vi "Metric.vi"(5 "Action":enum16{"Init", "Check"}(ring)) -> (2 "Metric?":bool)   [LabVIEW 2011]
uses:
  Globals/SysGlbs.vi
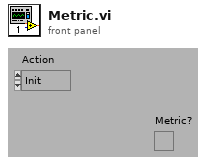
[diagram p1: front panel]
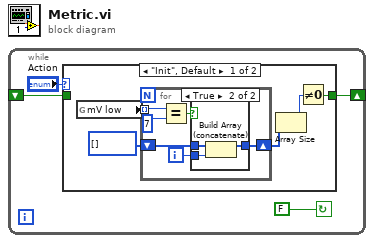
[diagram p0: block diagram]
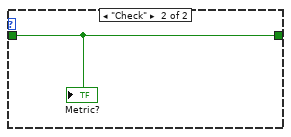
[diagram p3: hidden frame]
diagram:
  n1 = while {
    shift-left: _ -> [w3]
    shift-right: [w4] -> _
    stop <- FALSE continue-if-true
    n2 = case shown="\"Init\", Default" "Action" {
      tunnel: [w6 w20] -> w4
      tunnel: w3 -> [_ w20]
      frame "Init", Default {
        n3 = global read "SysGlbs.vi" "mV low"() -> (w8:i32[])
        n4 = for {
          shift-right: [w11] -> w5
          shift-left: i32[] [] ("Array Constant") -> [w12]
          tunnel: w8 -> [w15] mode=indexing
          i -> [w10]
          n5 = Equal?(x=w15, y=7) -> (x = y?=w13:bool)
          n6 = case shown="True" w13 {
            tunnel: w12 -> [w16 w19]
            tunnel: [w16 w18] -> w11
            tunnel: w10 -> [_ w17]
            frame False {
            }
            frame True {
              n7 = Build Array (concatenate)(w19, w17) -> (w18:i32[])
            }
          }
        }
        n8 = Array Size(array=w5) -> (size(s)=w7:i32)
        n9 = Not Equal To 0?(x=w7) -> (x != 0?=w6:bool)
      }
      frame "Check" {
        "Metric?" <- w20
      }
    }
  }
